vi "Get Self Event Registration.vi"(11 "Mediated Actor in":refnum<class "Mediated Actor.lvclass">) -> (2 "Event Registration Refnum":refnum<event-registration>, 3 "Mediated Actor out":refnum<class "Mediated Actor.lvclass">)   [LabVIEW 2016, in "Stream Mediator.lvlib" / "Mediated Actor.lvclass"]
doc: "--\nCopyright © 2017 Composed SystemsI All rights reserved.\n\nAuthor: Jon McBee <jon.mcbee@composed.io>\n\nThis library is provided \"AS IS\" ,WITHOUT WARRANTIES OR\nCONDITIONS OF ANY KIND, either express or implied.\n\nComposed Systems -- composed.io\n\nStream 0.0.1.1\nJon McBee - Composed Systems\nCopyright (c) 2017, Composed Systems"
uses:
  <userlib>/Composed Systems/Stream/Mediator/Classes/Mediated Actor/Mediated Actor.lvclass
  <userlib>/Composed Systems/Stream/Mediator/Classes/Message Interface/Message Interface.lvclass
  <userlib>/Composed Systems/Stream/Mediator/Classes/Mediated Actor/Mediated Actor.lvclass/Mediated Actor.ctl
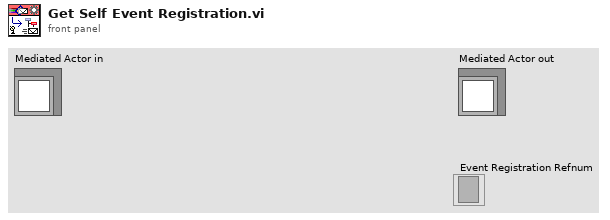
[diagram p1: front panel]
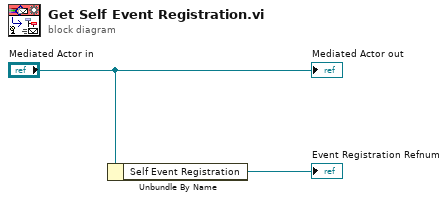
[diagram p0: block diagram]
diagram:
  n1 = Unbundle By Name("Mediated Actor in") -> ("Self Event Registration"=→"Event Registration Refnum":refnum<event-registration>)
  "Mediated Actor out" <- "Mediated Actor in"
